vi "get_status.vi"(8 "error in (no error)":errorcluster, 11 "GenericEmissionSensor.lvclass in":refnum<class "GenericDetector.lvclass">) -> (0 "error out":errorcluster, 2 "status":T1, 3 "GenericEmissionSensor.lvclass out":refnum<class "GenericDetector.lvclass">)   [LabVIEW 2010, in "GenericDetector.lvclass"]
uses:
  GenericDetector.lvclass
  status_enum.ctl
  GenericDetector.lvclass/GenericDetector.ctl
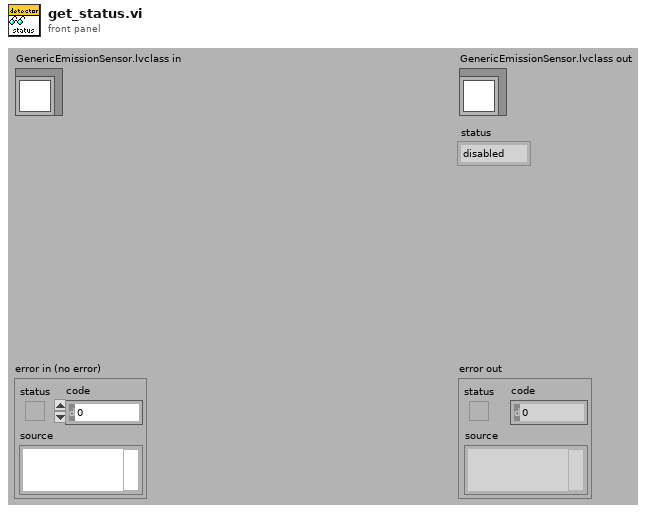
[diagram p1: front panel]
types:
  T1 = typedef "GenericDetector.lvclass/status_enum.ctl" = enum16{"disabled", "enabled"}
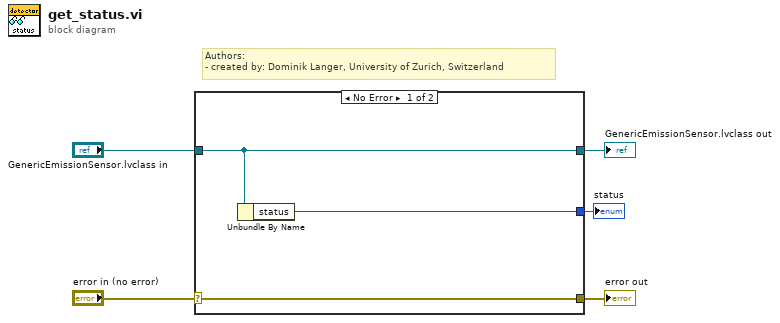
[diagram p0: block diagram]
diagram:
  # "Authors: \n- created by: Dominik Langer, University of Zurich, Switzerland"
  n1 = case shown="No Error" "error in (no error)" {
    selector: "error in (no error)" -> [w8 w9]
    tunnel: [w8 w9] -> w4
    tunnel: [w7 w10] -> w2
    tunnel: "GenericEmissionSensor.lvclass in" -> [w7 w10]
    tunnel: [w6 _] -> w1
    frame No Error {
      n2 = Unbundle By Name(w7) -> ("status"=w6:T1)
    }
    frame Error {
    }
  }
  "error out" <- w4
  "GenericEmissionSensor.lvclass out" <- w2
  "status" <- w1
